vi "File Dialog.vi"(7 "Prompt":refnum<class "UTF-8 String.lvclass">, 8 "error in":errorcluster) -> (0 "error out":errorcluster, 1 "Cancelled":bool, 3 "Selected Path":refnum<class "UTF-8 Path.lvclass">)   [LabVIEW 2020, in "G-Unicode.lvlib"]
uses:
  G-Unicode.lvlib
  Types/UTF-8 String/UTF-8 String.lvclass
  Types/UTF-8 Path/UTF-8 Path.lvclass
  Types/UTF-8 String/UTF-8 String.lvclass/UTF-8 String.ctl
  Types/UTF-8 Path/UTF-8 Path.lvclass/UTF-8 Path.ctl
  5e45d823-9f68-409d-aa25-7171c1de3c4c.vi
  9afeabe8-8abe-4536-bea1-05e5a3549c28.vi
  Types/UTF-8 String/Read Raw UTF-8 String.vi
  9afeabe8-8abe-4536-bea1-05e5a3549c28.vi/fad528d8-0ab0-4386-b479-4ccb3289bfd4.vi
  Types/UTF-8 Path/Write Raw UTF-8 Path.vi
  lib/g_unicode_32.dll
panel:
  out "array":string[](array[string])
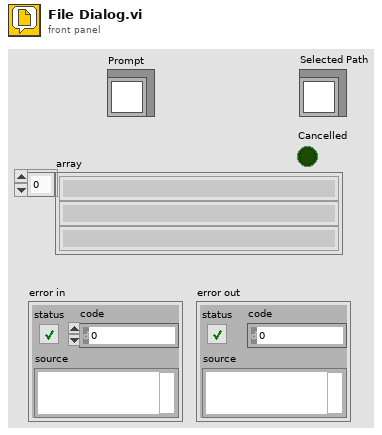
[diagram p1: front panel]
types:
  T1 = typedef "G-Unicode.lvlib/Raw UTF-8 String.ctl" = string
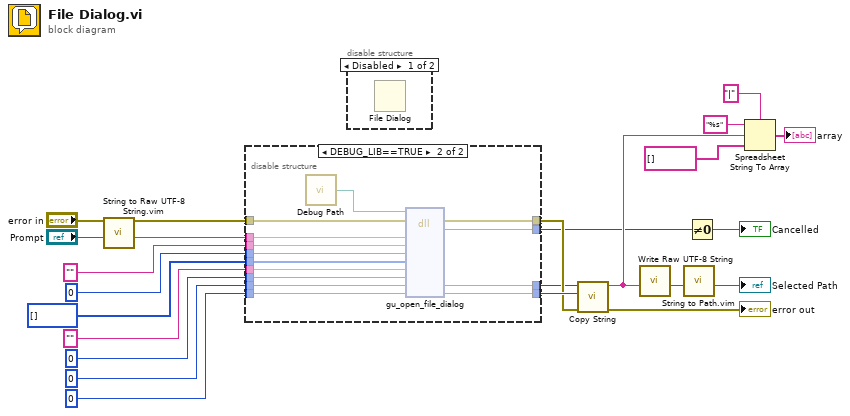
[diagram p0: block diagram]
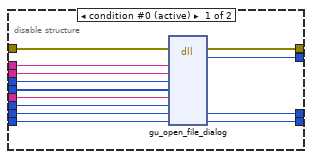
[diagram p3: hidden frame]
diagram:
  n1 = call "String to Raw UTF-8 String.vim"("error in"="error in", "String"="Prompt") -> ("Raw UTF-8 String"=w20:T1, "error out"=w12:errorcluster)  [unwired: 8 in]
  n2 = disable-structure shown="DEBUG_LIB==TRUE" {
    disable-tunnel: w12 -> [w37 w51]
    disable-tunnel: [w36 w50] -> w5
    disable-tunnel: w20 -> [w35 w49]
    disable-tunnel: "" ("default_path") -> [w34 w48]
    disable-tunnel: 0 ("num_filter_patterns") -> [w33 w47]
    disable-tunnel: i64[] [] ("filter_patterns") -> [w32 w46]
    disable-tunnel: "" ("filter_description") -> [w31 w45]
    disable-tunnel: 0 ("allow_multi_select") -> [w30 w44]
    disable-tunnel: i64 0 ("path_pointer") -> [w29 w43]
    disable-tunnel: 0 ("path_length") -> [w28 w42]
    disable-tunnel: [w27 w41] -> w1
    disable-tunnel: [w26 w40] -> w7
    disable-tunnel: [w25 w39] -> w4
    frame condition #0 (active) {
      n3 = dll-call lib="C:/github/dataflowg/g-unicode/src/LabVIEW/G-Unicode/lib/g_unicode_*.*" fn="gu_open_file_dialog"(error in=w37, "title"=w35, "default_path"=w34, "num_filter_patterns"=w33, "filter_patterns"=w32, "filter_description"=w31, "allow_multi_select"=w30, "path_pointer"=w29, "path_length"=w28) -> (error out=w36:errorcluster, "return type"=w25:i32, "path_pointer"=w27:i64, "path_length"=w26:i32)  [unwired: 8 in, 1 out]
    }
    frame condition #1 {
      n4 = call "Debug Path.vi"() -> ("Debug Path"=w38:path)
      n5 = dll-call lib="?" fn="gu_open_file_dialog"(path in=w38, error in=w51, "title"=w49, "default_path"=w48, "num_filter_patterns"=w47, "filter_patterns"=w46, "filter_description"=w45, "allow_multi_select"=w44, "path_pointer"=w43, "path_length"=w42) -> (error out=w50:errorcluster, "return type"=w39:i32, "path_pointer"=w41:i64, "path_length"=w40:i32)  [unwired: 7 in, 1 out]
    }
  }
  n6 = disable-structure shown="Disabled" {
    frame Disabled {
      n7 = File Dialog() -> ()  [unwired: 7 in, 4 out]
    }
    frame Enabled {
    }
  }
  n8 = call "Copy String.vi"("error in"=w5, "size"=w7, "pointer"=w1) -> ("error out"=→"error out":errorcluster, "string"=w6:string)  [unwired: 7 in]
  n9 = call "Write Raw UTF-8 String.vi"("Raw UTF-8 String"=w6) -> ("UTF-8 String"=w11:refnum<class "UTF-8 String.lvclass">)  [unwired: 10 in]
  n10 = call "String to Path.vim"("String"=w11) -> ("Path"=→"Selected Path":refnum<class "UTF-8 Path.lvclass">)  [unwired: 9 in, 1 out]
  n11 = Not Equal To 0?(x=w4) -> (x != 0?=→"Cancelled":bool)
  n12 = Spreadsheet String To Array(delimiter (Tab)="|", format string="%s", spreadsheet string=w6, array type (2D Dbl)=string[] []) -> (array=→"array":string[])
